vi "ConvertTo(DBL).vi"(8 "error in":errorcluster, 9 "Message Payload":variant) -> (0 "error out":errorcluster, 1 "Message Payload DBL Numeric":dbl)   [LabVIEW 2018]
doc: "Convert variant to DBL scalar\n\nBolder Software LLC"
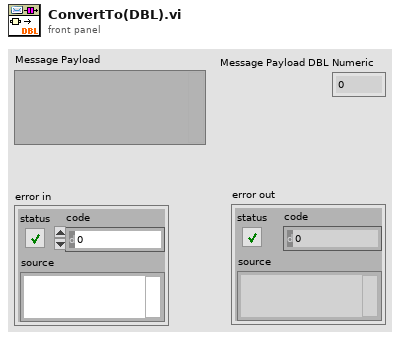
[diagram p1: front panel]
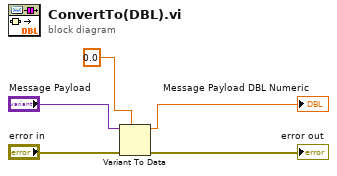
[diagram p0: block diagram]
diagram:
  n1 = Variant To Data(error in="error in", type=0.0 ("Message Payload DBL Numeric"), Variant="Message Payload") -> (data=→"Message Payload DBL Numeric":dbl, error out=→"error out":errorcluster)
